vi "ZCAN_CloseDevice.vi"(8 "error in (no error)":errorcluster caption="错误输入（无错误）", 10 "device_handle":u32) -> (0 "error out":errorcluster caption="错误输出", 2 "Close_success?":bool)   [LabVIEW 2018]
doc: "该函数用于关闭设备，关闭设备和打开设备一一对应。\n\n调用该函数，会关闭整个CAN设备（对于设备句柄），不分通道。"
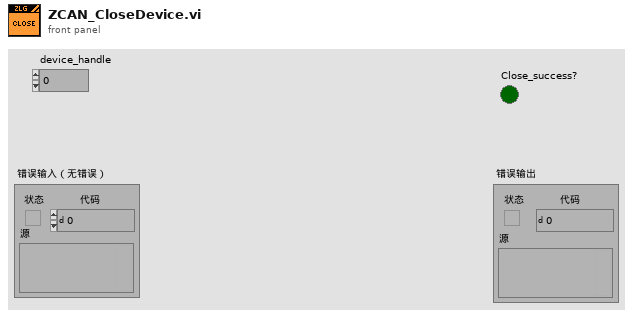
[diagram p1: front panel]
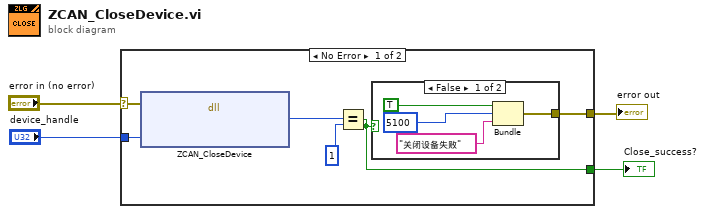
[diagram p0: block diagram]
diagram:
  n1 = case shown="No Error" "error in (no error)" {
    selector: "error in (no error)" -> [w5 w15]
    tunnel: [w8 w15] -> w3
    tunnel: "device_handle" -> [w10 _]
    tunnel: [w6 _] -> w1
    frame No Error {
      n2 = dll-call lib="PTH2tabs CUsersadminDesktop\"2020版本 zlgcan_labview_20220510zlgcan_demo_PCIECANFD-200Ubinzlgcan_wrap.dll" fn="ZCAN_CloseDevice" ("ZCAN_StartCAN")(error in=w5, "device_handle"=w10) -> ("return"=w7:u32)  [unwired: 3 in, 2 out]
      n3 = Equal?(x=w7, y=1) -> (x = y?=w6:bool)
      n4 = case shown="False" w6 {
        tunnel: [w11 _] -> w8
        frame False {
          n5 = Bundle("status"=TRUE, "code"=5100, "消息"="关闭设备失败") -> (w11:cluster{"status":bool, "code":i32, "消息":string})  [unwired: 1 in]
        }
        frame True {
        }
      }
    }
    frame Error {
    }
  }
  "error out" <- w3
  "Close_success?" <- w1
